vi "getScriptList.vi"(8 "error in (no error)":errorcluster, 11 "MatlabScripts in":refnum<class "MatlabScripts.lvclass">) -> (0 "error out":errorcluster, 2 "scriptNames":string[](array[string]), 3 "MatlabScripts out":refnum<class "MatlabScripts.lvclass">)   [LabVIEW 2011, in "Views.lvlib" / "ExperimentControl.lvlib" / "MatlabScripts.lvclass"]
uses:
  MatlabScripts.lvclass
  Tools/Filing/FileSystem/FileSystem.lvclass
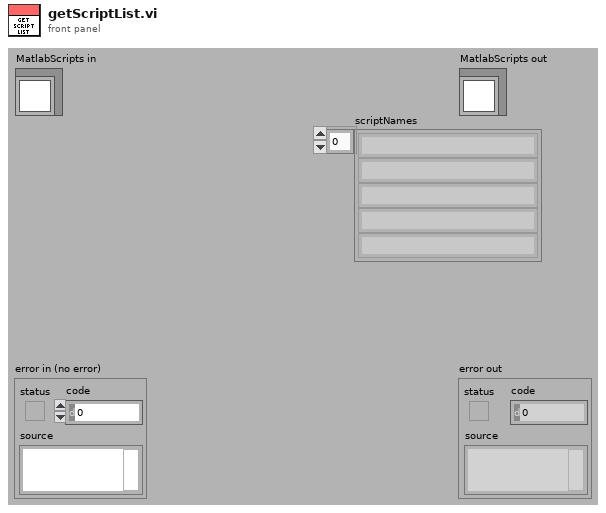
[diagram p1: front panel]
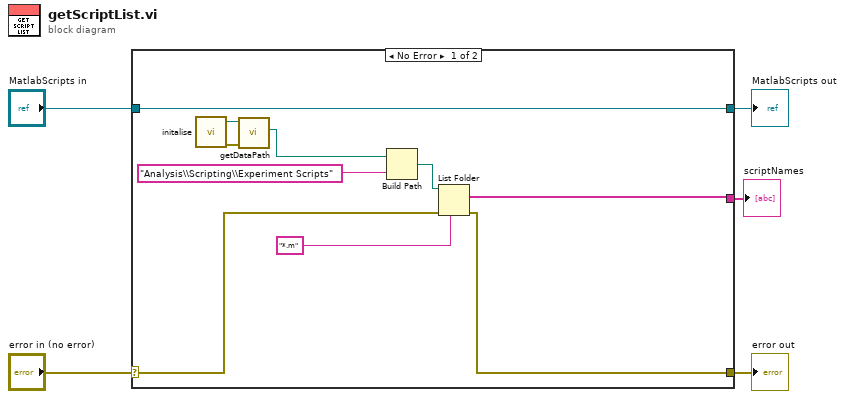
[diagram p0: block diagram]
diagram:
  n1 = case shown="No Error" "error in (no error)" {
    selector: "error in (no error)" -> [w13 w17]
    tunnel: [w12 w17] -> w4
    tunnel: [w15 w16] -> w2
    tunnel: "MatlabScripts in" -> [w15 w16]
    tunnel: [w11 _] -> w1
    frame No Error {
      n2 = call "initalise.vi"() -> ("error out"=w8:errorcluster, "FileSystem out"=w7:refnum<class "FileSystem.lvclass">)  [unwired: 10 in]
      n3 = call-dynamic "getDataPath.vi"("error in (no error)"=w8, "FileSystem.lvclass in"=w7) -> ("DataPath"=w6:path)  [unwired: 7 in, 2 out]
      n4 = Build Path(base path=w6, name or relative path="Analysis\\Scripting\\Experiment Scripts") -> (appended path=w10:path)
      n5 = List Folder(path=w10, pattern="*.m", error in=w13) -> (filenames=w11:string[], error out=w12:errorcluster)  [unwired: 1 in, 2 out]
    }
    frame Error {
    }
  }
  "error out" <- w4
  "MatlabScripts out" <- w2
  "scriptNames" <- w1
